vi "GlobalFan2.vi"() -> ()   [LabVIEW 2024]
panel:
  out "Fan2":bool
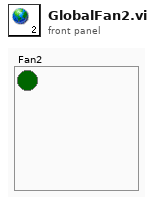
[diagram p1: front panel]
diagram:
